vi "REPORT_PBATCH_filter_records.vi"(9 "REPORT_DATES_filters":T1={"order_selection"=enum."new_to_old", "last_OP"="", "last_status"=""}, 10 "gear_statuses":T2[](array[typedef]), 11 "gears":string[][](array[string])) -> (2 "record_statuses":T2[](array[typedef]), 3 "ItemNames":string[][](array[string]))   [LabVIEW 2019]
uses:
  DATES/typedef/REPORT_DATES_statuses.ctl
  typedef/REPORT_PBATCH_filters.ctl
  <userlib>/_OpenG.lib/array/array.llb/Reverse 2D Array (String)__ogtk.vi
  <userlib>/_OpenG.lib/array/array.llb/Filter 1D Array with Scalar (String)__ogtk.vi
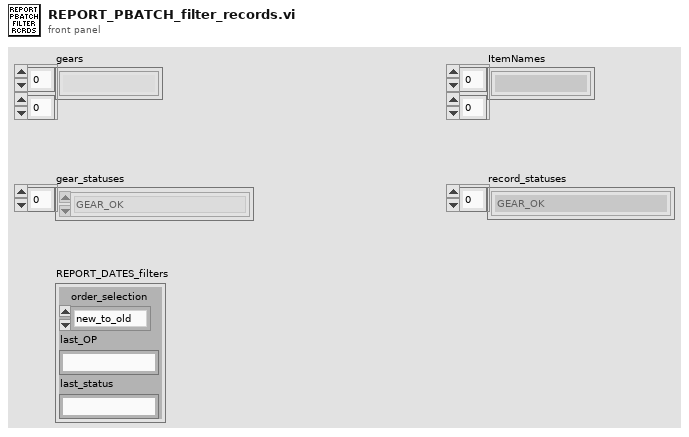
[diagram p1: front panel]
types:
  T1 = typedef "REPORT_PBATCH_filters.ctl" = cluster{"order_selection":enum32{"old_to_new", "new_to_old"}, "last_OP":string, "last_status":string}
  T2 = typedef "REPORT_DATES_statuses.ctl" = enum16{"GEAR_OK", "GEAR_NOK", "GEAR_interrupted", "GEAR_in_operation", "GEAR_unexpected"}
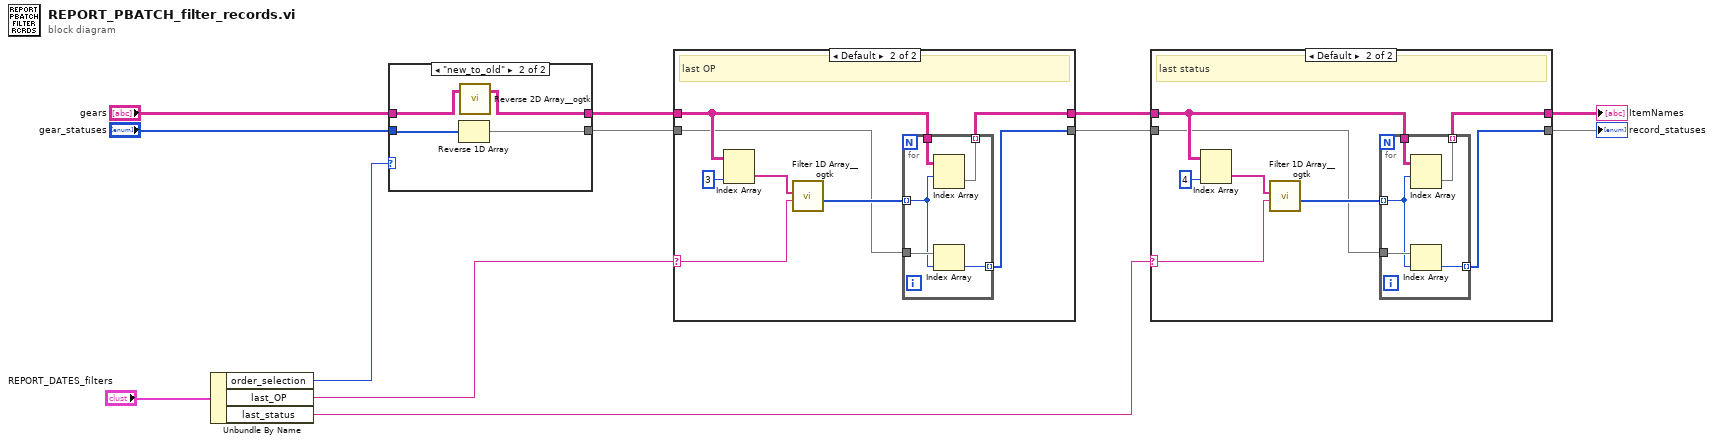
[diagram p0: block diagram]
diagram:
  n1 = Unbundle By Name("REPORT_DATES_filters") -> ("order_selection"=w9:enum32{"old_to_new", "new_to_old"}, "last_OP"=w8:string, "last_status"=w1:string)
  n2 = case shown="\"new_to_old\"" w9 {
    tunnel: "gears" -> [w14 w16]
    tunnel: [w14 w15] -> w7
    tunnel: "gear_statuses" -> [w13 w18]
    tunnel: [w13 w17] -> w6
    frame "old_to_new" {
    }
    frame "new_to_old" {
      n3 = Reverse 1D Array(array=w18) -> (reversed array=w17:T2[])
      n4 = call-poly <userlib>:"Reverse 2D Array__ogtk.vi"("Array"=w16) -> ("Reversed Array"=w15:string[][])  [unwired: 2 in]
    }
  }
  n5 = case shown="Default" w8 {
    selector: w8 -> [_ w28]
    tunnel: [w20 w25] -> w5
    tunnel: w7 -> [w20 w23]
    tunnel: w6 -> [w19 w22]
    tunnel: [w19 w21] -> w4
    frame "ALL" {
      # "last OP"
    }
    frame Default {
      # "last OP"
      n6 = Index Array(array=w23, index (col)=3 ("disabled index (col)")) -> (element=w26:string[])  [unwired: 1 in]
      n7 = call-poly <userlib>:"Filter 1D Array__ogtk.vi"("items to filter"=w28, "array"=w26) -> ("filtered item indices"=w24:i32[])  [unwired: 4 in, 1 out]
      n8 = for {
        tunnel: w23 -> [w33]
        tunnel: w24 -> [w30] mode=indexing
        tunnel: [w32] -> w25 mode=indexing
        tunnel: w22 -> [w31]
        tunnel: [w29] -> w21 mode=indexing
        n9 = Index Array(array=w33, index (row)=w30) -> (element=w32:string[])  [unwired: 1 in]
        n10 = Index Array(array=w31, index=w30) -> (element=w29:T2)
      }
    }
  }
  n11 = case shown="Default" w1 {
    selector: w1 -> [_ w43]
    tunnel: [w35 w40] -> w3
    tunnel: w5 -> [w35 w38]
    tunnel: w4 -> [w34 w37]
    tunnel: [w34 w36] -> w2
    frame "ALL" {
      # "last status"
    }
    frame Default {
      # "last status"
      n12 = Index Array(array=w38, index (col)=4 ("disabled index (col)")) -> (element=w41:string[])  [unwired: 1 in]
      n13 = call-poly <userlib>:"Filter 1D Array__ogtk.vi"("items to filter"=w43, "array"=w41) -> ("filtered item indices"=w39:i32[])  [unwired: 4 in, 1 out]
      n14 = for {
        tunnel: w38 -> [w48]
        tunnel: w39 -> [w45] mode=indexing
        tunnel: [w47] -> w40 mode=indexing
        tunnel: w37 -> [w46]
        tunnel: [w44] -> w36 mode=indexing
        n15 = Index Array(array=w48, index (row)=w45) -> (element=w47:string[])  [unwired: 1 in]
        n16 = Index Array(array=w46, index=w45) -> (element=w44:T2)
      }
    }
  }
  "ItemNames" <- w3
  "record_statuses" <- w2
